vi "WriteSharedVariables_org.vi"() -> ()   [LabVIEW 2014]
uses:
  <vilib>/Platform/TimedLoop/XDataNode/timing_clust.ctl
  <vilib>/Platform/TimedLoop/XDataNode/nitl_modes.ctl
  <vilib>/Platform/TimedLoop/XDataNode/wakeup.ctl
  <vilib>/platform/TimedLoop/XDataNode/XDataNode.xnode
  <vilib>/Platform/TimedLoop/XDataNode/XDNodeRunTimeDep.lvlib
panel:
  in  "no. Variables":i32=1000
  out "Slide":i32(slide) max=100 scale=0.0..1000.0
  out "B1 3":bool
  out "B1 2":bool
  out "B1":bool
  out "Delays":u64
  out "Counter":i32
  in  "error in":errorcluster
  in  "stop 2":bool
  in  "stop":bool
  in  "Run Time (ms)":i32=100
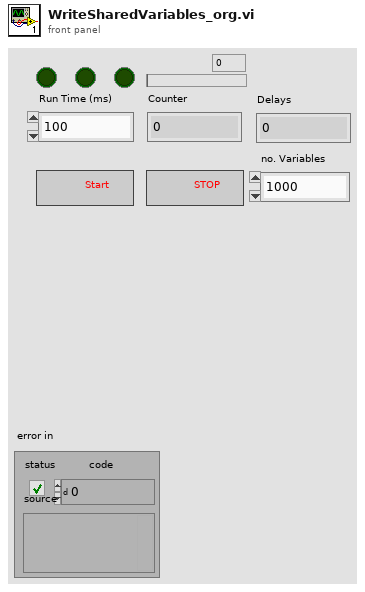
[diagram p1: front panel]
types:
  T1 = cluster{"Number of Variables":i32, "Variable/Parent Name array":string[][], "URL array":string[], "Type array":string[]}
  T2 = typedef "XDNodeRunTimeDep.lvlib/timing_clust.ctl" = cluster{"Expected End [f-1]":u64, "Actual End [f-1]":u64, "Finished Late? [f-1]":bool, "Expected End [i-1]":u64, "Actual End [i-1]":u64, "Finished Late? [i-1]":bool, "Expected Start [i]":u64, "Actual Start [i]":u64, "Expected Start [f]":u64, "Actual Start [f]":u64, "Source Name":string, "Structure Name":string, "Period":i64, "Deadline":i64, "Offset":i64, "Start":i64, "Priority":i32, "Timeout":i32, "Mode":T3, "Wakeup Reason":T4, "Error":errorcluster, "Source Type":string, "Secondary Source Type":string, "Global End Time":u64, "Global Start Time":u64, "Frame Duration":u64, "Iteration Duration":u64, "Assigned CPU":i32, "I/O Scan Engine Mode":u32}
  T3 = typedef "XDNodeRunTimeDep.lvlib/nitl_modes.ctl" = enum32{"No Change", "Process missed periods, maintain original phase", "Discard missed periods, maintain original phase", "Process missed periods, ignore original phase", "Discard missed periods, ignore original phase"}
  T4 = typedef "XDNodeRunTimeDep.lvlib/wakeup.ctl" = enum32{"Normal", "Aborted", "Asynchronous wakeup", "Timing source error", "Timed loop error", "Timeout"}
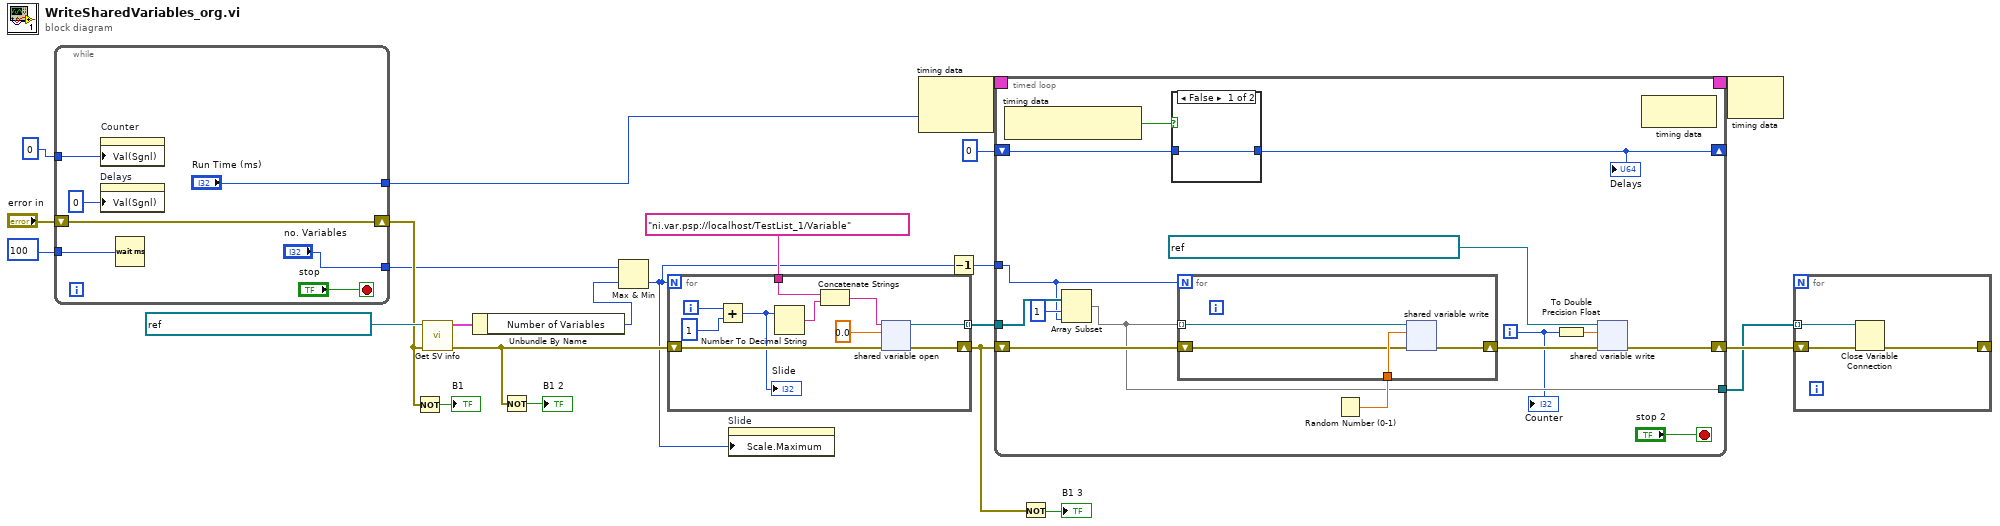
[diagram p0: block diagram]
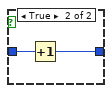
[diagram p2: hidden frame]
diagram:
  n1 = while {
    tunnel: ["Run Time (ms)"] -> w21
    shift-right: [w29] -> w12
    shift-left: "error in" -> [w29]
    tunnel: u32 100 ("milliseconds to wait") -> [w28]
    tunnel: 0 ("milliseconds to wait") -> [w27]
    tunnel: ["no. Variables"] -> w4
    stop <- "stop" stop-if-true
    n2 = property on="Counter" class="DigNum (strict)"("Val(Sgnl)"=w27) -> ()  [unwired: 2 in, 2 out]
    n3 = property on="Delays" class="DigNum (strict)"("Val(Sgnl)"=u64 0 ("Value (Signaling)")) -> ()  [unwired: 2 in, 2 out]
    n4 = Wait (ms)(milliseconds to wait=w28) -> ()  [unwired: 1 out]
  }
  n5 = Not(x=w12) -> (.not. x?=→"B1":bool)
  n6 = call "Get SV info.vi"("Error In"=w12, "container refnum in"=refnum<k21> "ni.var.psp://localhost/TestList_1") -> ("Error Out"=w11:errorcluster, "Deployed Shared Variable Information"=w15:T1)  [unwired: 7 in, 1 out]
  n7 = Unbundle By Name(w15) -> ("Number of Variables"=w6:i32)
  n8 = Not(x=w11) -> (.not. x?=→"B1 2":bool)
  n9 = Max & Min(x=w4, y=w6) -> (min(x,y)=w5:i32)  [unwired: 1 out]
  n10 = for {
    N: w5 -> [_]
    shift-right: [w37] -> w8
    shift-left: w11 -> [w36]
    tunnel: "ni.var.psp://localhost/TestList_1/Variable" -> [w35]
    tunnel: [w31] -> w2 mode=indexing
    i -> [w33]
    n11 = Add(x=w33, y=1) -> (x+y=w32:i32)
    "Slide" <- w32
    n12 = Number To Decimal String(number=w32) -> (decimal integer string=w40:string)  [unwired: 1 in]
    n13 = Concatenate Strings(w35, w40) -> (w38:string)
    n14 = shared-variable-open(w38, w36, 0.0) -> (w31:refnum<k21>, w37:errorcluster)  [unwired: 1 in]
  }
  n15 = property on="Slide" class="Slide (strict)"("Scale.Maximum"=w5) -> ()  [unwired: 2 in, 2 out]
  n16 = node-c288(w21) -> (w23:T2)  [unwired: 1 in]
  n17 = Decrement(x=w5) -> (x-1=w14:i32)
  n18 = timed-loop {
    timing: w23 -> [_]
    timing-out: [_] -> w22
    shift-right: [w52] -> w3
    shift-left: w8 -> [w51]
    shift-right: [w47] -> _
    shift-left: u64 0 -> [w48]
    tunnel: w14 -> [w44]
    tunnel: w2 -> [w46]
    tunnel: [w43] -> w1
    i -> [w41]
    stop <- "stop 2" stop-if-true
    n19 = node-c288() -> (w49:bool)  [unwired: 1 in]
    n20 = Array Subset(array=w46, index=1, length=w44) -> (w43:refnum<k21>[])
    n21 = case shown="False" w49 {
      tunnel: w48 -> [w56 w58]
      tunnel: [w56 w57] -> w47
      frame False {
      }
      frame True {
        n22 = Increment(x=w58) -> (x+1=w57:u64)
      }
    }
    "Delays" <- w47
    n23 = Random Number (0-1)() -> (number: 0 to 1=w55:dbl)
    n24 = for {
      N: w44 -> [_]
      tunnel: w55 -> [w62]
      shift-right: [w61] -> w54
      shift-left: w51 -> [w60]
      tunnel: w43 -> [w59] mode=indexing
      n25 = shared-variable-write(w59, w60, w62) -> (w61:errorcluster)  [unwired: 1 out]
    }
    n26 = To Double Precision Float(number=w41) -> (double precision float=w42:dbl)
    n27 = shared-variable-write(refnum<k21> "ni.var.psp://localhost/TestList_1/Variable1" ("shared variable refnum in"), w54, w42) -> (w52:errorcluster)  [unwired: 1 out]
    n28 = node-c288() -> ()  [unwired: 1 in, 1 out]
    "Counter" <- w41
  }
  n29 = Not(x=w8) -> (.not. x?=→"B1 3":bool)
  n30 = node-c288(w22) -> ()  [unwired: 1 out]
  n31 = for {
    shift-right: [w66] -> _
    shift-left: w3 -> [w68]
    tunnel: w1 -> [w67] mode=indexing
    n32 = Close Variable Connection(8:w68, 11:w67) -> (0:w66:errorcluster)
  }
